vi "SLL DE List all Global Virtual Channels from MAX v2.vi"(8 "error in (no error)":errorcluster) -> (0 "error out":errorcluster, 2 "Analog Output":refnum<k21>[](array[refnum]), 3 "Analog Input":refnum<k21>[](array[refnum]), 4 "Digital Output":refnum<k21>[](array[refnum]), 5 "Digital Input":refnum<k21>[](array[refnum]), 6 "Counter Output":refnum<k21>[](array[refnum]), 7 "Counter Input":refnum<k21>[](array[refnum]))   [LabVIEW 2013]
doc: "This VI will list 'Virtual Global Channels' from MAX.\nAlso seperates these channels based on AIO, DIO and CIO (Channel type or catagory)\n\nCopyright © 2009, Soliton Technologies.\nAll rights reserved."
uses:
  <resource>/objmgr/daqmx.rc
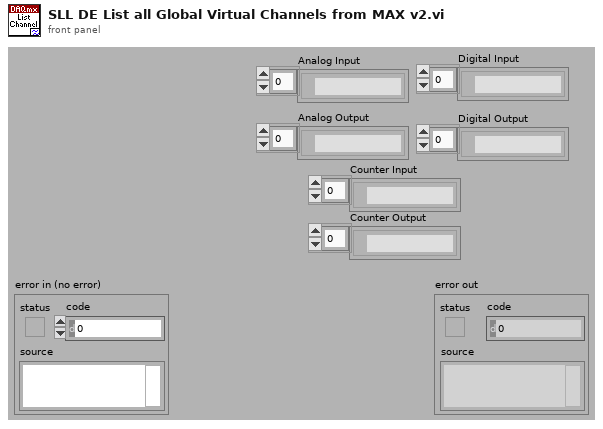
[diagram p1: front panel]
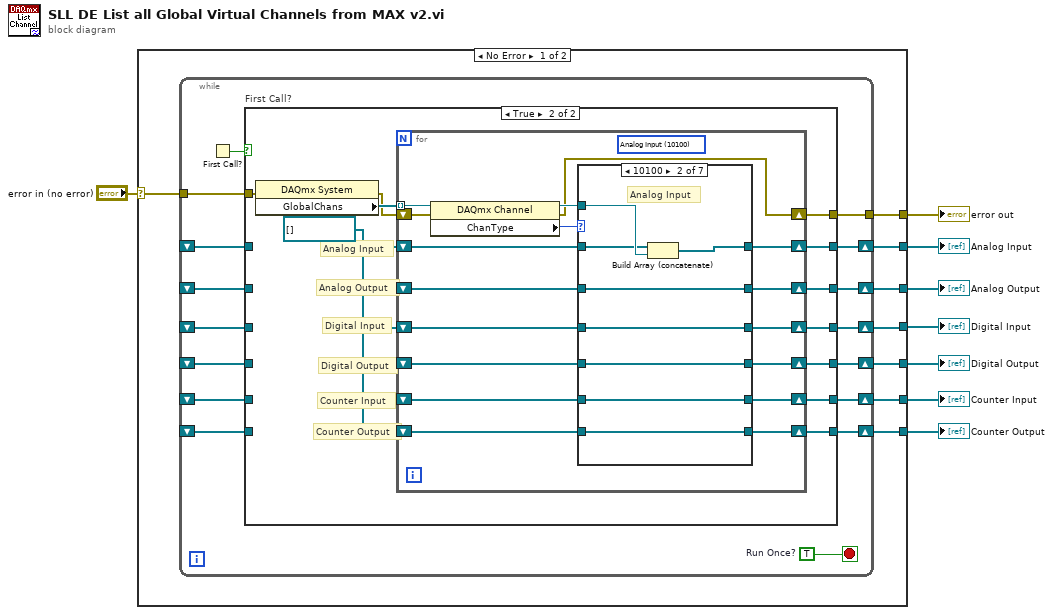
[diagram p0: block diagram]
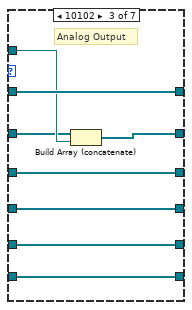
[diagram p4: hidden frame]
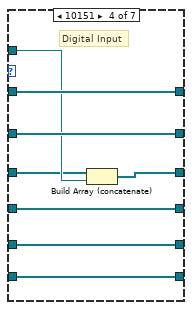
[diagram p5: hidden frame]
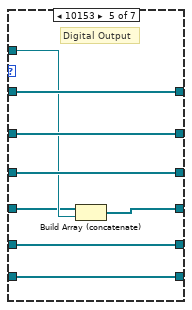
[diagram p6: hidden frame]
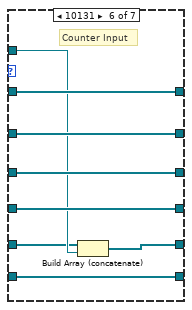
[diagram p7: hidden frame]
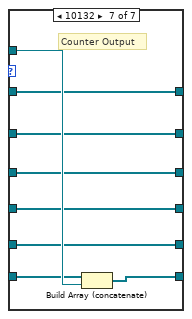
[diagram p8: hidden frame]
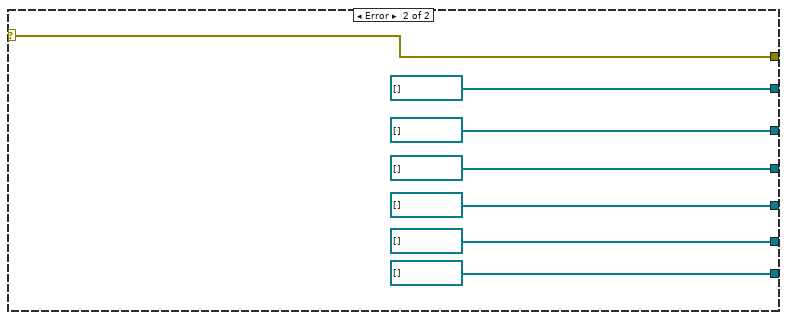
[diagram p9: hidden frame]
diagram:
  n1 = case shown="No Error" "error in (no error)" {
    selector: "error in (no error)" -> [w16 w128]
    tunnel: [w15 refnum<k21>[] []] -> w7
    tunnel: [w14 refnum<k21>[] []] -> w6
    tunnel: [w13 refnum<k21>[] []] -> w5
    tunnel: [w12 refnum<k21>[] []] -> w4
    tunnel: [w11 refnum<k21>[] []] -> w3
    tunnel: [w10 refnum<k21>[] []] -> w2
    tunnel: [w9 w128] -> w1
    frame No Error {
      n2 = while {
        tunnel: w16 -> [w31]
        shift-right: [w24] -> w10
        shift-left: _ -> [w18]
        shift-right: [w25] -> w11
        shift-left: _ -> [w19]
        shift-right: [w26] -> w12
        shift-left: _ -> [w20]
        shift-right: [w27] -> w13
        shift-left: _ -> [w21]
        shift-right: [w28] -> w14
        shift-left: _ -> [w22]
        shift-right: [w29] -> w15
        shift-left: _ -> [w23]
        tunnel: [w17] -> w9
        stop <- w32 stop-if-true
        w32 = TRUE  # Run Once?
        n3 = First Call?() -> (First Call?: T/F=w30:bool)
        n4 = case "First Call?" shown="True" w30 {
          tunnel: w31 -> [w33 w50]
          tunnel: [w39 w47] -> w29
          tunnel: [w38 w46] -> w28
          tunnel: [w37 w45] -> w27
          tunnel: [w36 w44] -> w26
          tunnel: [w35 w43] -> w25
          tunnel: [w34 w42] -> w24
          tunnel: w23 -> [w39 _]
          tunnel: w22 -> [w38 _]
          tunnel: w21 -> [w37 _]
          tunnel: w20 -> [w36 _]
          tunnel: w19 -> [w35 _]
          tunnel: w18 -> [w34 _]
          tunnel: [w33 w41] -> w17
          frame False {
          }
          frame True {
            w40 = refnum<k21>[] []
            # "Analog Input"
            # "Analog Output"
            # "Digital Input"
            # "Digital Output"
            # "Counter Input"
            # "Counter Output"
            n5 = property class="DAQmx System"(error in=w50) -> (error out=w48:errorcluster, "GlobalChans"=w49:refnum<k21>[])  [unwired: 1 in, 1 out]
            n6 = for {
              tunnel: w49 -> [w67] mode=indexing
              shift-right: [w63] -> w47
              shift-left: w40 -> [w62]
              shift-right: [w61] -> w46
              shift-left: w40 -> [w60]
              shift-right: [w59] -> w45
              shift-left: w40 -> [w58]
              shift-right: [w57] -> w44
              shift-left: w40 -> [w56]
              shift-right: [w55] -> w43
              shift-left: w40 -> [w54]
              shift-right: [w53] -> w42
              shift-left: w40 -> [w52]
              shift-right: [w51] -> w41
              shift-left: w48 -> [w66]
              (unwired) 10100 items=["Analog Input"=10100, "Analog Output"=10102, "Digital Input"=10151, "Digital Output"=10153, "Counter Input"=10131, "Counter Output"=10132] ("ChanType")
              n7 = property class="DAQmx Channel"(reference=w67, error in=w66) -> (reference out=w64:refnum<k21>, error out=w51:errorcluster, "ChanType"=w65:i32)
              n8 = case shown="10100" w65 {
                tunnel: w64 -> [_ w81 w88 w95 w102 w108 w121]
                tunnel: [w73 w80 w89 w97 w105 w113 w114] -> w63
                tunnel: w62 -> [w73 w79 w89 w97 w105 w113 w114]
                tunnel: [w72 w78 w87 w96 w104 w112 w115] -> w61
                tunnel: w60 -> [w72 w78 w86 w96 w104 w112 w115]
                tunnel: [w71 w77 w85 w94 w103 w111 w116] -> w59
                tunnel: w58 -> [w71 w77 w85 w93 w103 w111 w116]
                tunnel: [w70 w76 w84 w92 w101 w110 w117] -> w57
                tunnel: w56 -> [w70 w76 w84 w92 w100 w110 w117]
                tunnel: [w69 w75 w83 w91 w99 w109 w118] -> w55
                tunnel: w54 -> [w69 w75 w83 w91 w99 w107 w118]
                tunnel: [w68 w74 w82 w90 w98 w106 w120] -> w53
                tunnel: w52 -> [w68 w74 w82 w90 w98 w106 w119]
                frame Default {
                }
                frame 10100 {
                  # "Analog Input"
                  n9 = Build Array (concatenate)(w79, w81) -> (w80:refnum<k21>[])
                }
                frame 10102 {
                  # "Analog Output"
                  n10 = Build Array (concatenate)(w86, w88) -> (w87:refnum<k21>[])
                }
                frame 10151 {
                  # "Digital Input"
                  n11 = Build Array (concatenate)(w93, w95) -> (w94:refnum<k21>[])
                }
                frame 10153 {
                  # "Digital Output"
                  n12 = Build Array (concatenate)(w100, w102) -> (w101:refnum<k21>[])
                }
                frame 10131 {
                  # "Counter Input"
                  n13 = Build Array (concatenate)(w107, w108) -> (w109:refnum<k21>[])
                }
                frame 10132 {
                  # "Counter Output"
                  n14 = Build Array (concatenate)(w119, w121) -> (w120:refnum<k21>[])
                }
              }
            }
          }
        }
      }
    }
    frame Error {
    }
  }
  "error out" <- w1
  "Analog Input" <- w7
  "Analog Output" <- w6
  "Digital Input" <- w5
  "Digital Output" <- w4
  "Counter Input" <- w3
  "Counter Output" <- w2
